vi "MAC_to_u32.vi"(11 "MAC (aa:bb:cc:dd:ee:ff)":u8[](array[numeric]) format="%02x") -> (2 "MSLW":u32 format="%.0x", 3 "LSLW":u32 format="%.0x")   [LabVIEW 2020, in "EthFrameManagement.lvlib"]
doc: "Convert MAC Address to Least Significant Longword (LSLW) and Most Significant Longword (MSLW) of the MAC Source Address."
uses:
  EthFrameManagement.lvlib
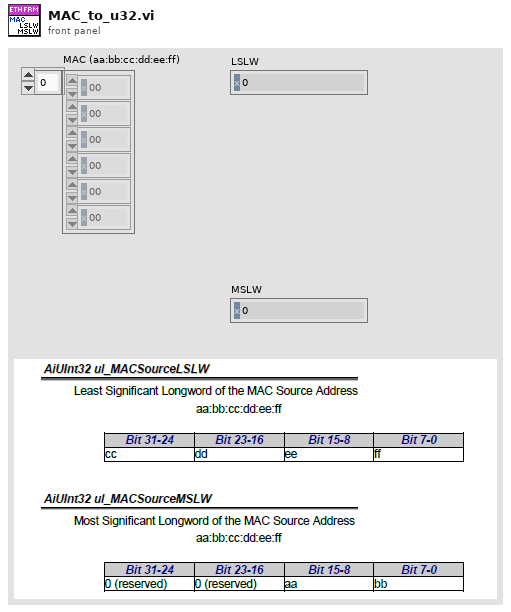
[diagram p1: front panel]
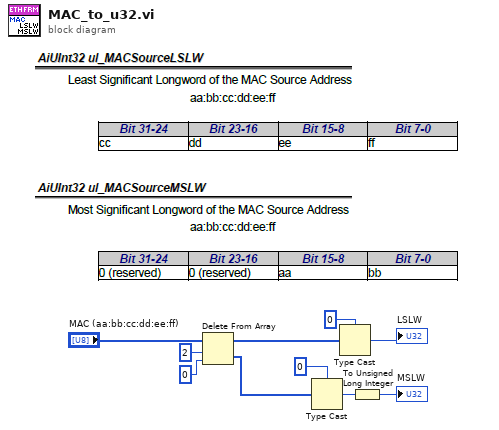
[diagram p0: block diagram]
diagram:
  n1 = Delete From Array(array="MAC (aa:bb:cc:dd:ee:ff)", length=2, index=0 ("length")) -> (deleted portion=w4:u8[], array with subset deleted=w3:u8[])
  n2 = Type Cast(type=u16 0 ("LSLW"), x=w4) -> (*(type *) &x=w2:u16)
  n3 = Type Cast(type=u32 0 ("LSLW"), x=w3) -> (*(type *) &x=→"LSLW":u32)
  n4 = To Unsigned Long Integer(number=w2) -> (unsigned 32bit integer=→"MSLW":u32)
